vi "Data retrieve engine_SE.vi"(0 "File or Folder Path":path=path "C:/Users/voodoo/Desktop/IV_separat_Vsgsweep_2fields_Vbg-2.8V", 5 "Scan names":string[](array[string]), 7 "IV setup":T3={"# of Vslow"=101, "# Vfast"=41, "#IV Curves at each gate"=1, "B/T offset"=0, "Discard first # curves"=0, "Manual offset"=0, "Field Period"=1, "# of fields/Temperatures"=1}, 9 "index":T2={"A"=3, "B"=4, "C"=2, "D"=4, "E"=3, "N1"=2, "N2"=2, "N3"=3, "N4"=4, "A 1"=8, "A 2"=14, "C 1"=5, "C 2"=1, "E 2"=4}, 11 "Portion of data":cluster{dbl, dbl}(slide)={0.75, 0.25} scale=0.0..1.0, 12 "Decimate point":dbl=1e-10 format="%#_1f", 13 "Extract paramaters from comments?":bool) -> (3 "Comments":string, 4 "IV":cluster{dbl[], dbl[]}[][](array[cluster])=[[{[-2.301174301585294e-09, -2.201174301585294e-09, -2.1011743015852944e-09, -2.0011743015852943e-09, -1.9011743015852942e-09, -1.8011743015852941e-09, -1.701174301585294e-09, -1.601174301585294e-09, -1.5011743015852941e-09, -1.401174301585294e-09, -1.301174301585294e-09, -1.2011743015852942e-09, -1.101174301585294e-09, -1.001174301585294e-09, -9.011743015852942e-10, -8.011743015852941e-10, -7.01174301585294e-10, -6.011743015852942e-10, -5.011743015852941e-10, -4.01174301585294e-10, -3.0117430158529395e-10, -2.0117430158529388e-10, -1.0117430158529423e-10, -1.1743015852941594e-12], [-2.4075285232756958e-05, -1.737972813858452e-05, -1.1037615852397166e-05, -5.267782040080203e-06, 2.4232289247411676e-07, 5.628820057942294e-06, 1.015781505747205e-05, 1.4463328409568988e-05, 1.817222828467457e-05, 2.105509970958606e-05, 2.409775741426245e-05, 2.720796229813868e-05, 3.0197002730537915e-05, 3.3043546244784785e-05, 3.5385544630750595e-05, 3.756777735485851e-05, 3.987253185589809e-05, 4.20620889081888e-05, 4.4006459573108544e-05, 4.587698979226302e-05, 4.7931581768717136e-05, 4.925252522526536e-05, 5.0480327825776546e-05, 8.08077413503745e-08]}]], 6 "IV-2T":cluster{dbl[], dbl[]}[][](array[cluster])=[[{[-2.301174301585294e-09, -2.201174301585294e-09, -2.1011743015852944e-09, -2.0011743015852943e-09, -1.9011743015852942e-09, -1.8011743015852941e-09, -1.701174301585294e-09, -1.601174301585294e-09, -1.5011743015852941e-09, -1.401174301585294e-09, -1.301174301585294e-09, -1.2011743015852942e-09, -1.101174301585294e-09, -1.001174301585294e-09, -9.011743015852942e-10, -8.011743015852941e-10, -7.01174301585294e-10, -6.011743015852942e-10, -5.011743015852941e-10, -4.01174301585294e-10, -3.0117430158529395e-10, -2.0117430158529388e-10, -1.0117430158529423e-10, -1.1743015852941594e-12], [-0.002353462043255516, -0.002297777119659299, -0.002239582947886705, -0.0021846959913649658, -0.0021298090348432263, -0.0020715829478867047, -0.0020166959913649656, -0.0019611544893886803, -0.0019081505368195105, -0.0018609817056506796, -0.0018106102770792509, -0.0017577829478867043, -0.001702609034843226, -0.001644382947886704, -0.001589759034843226, -0.001532834880253854, -0.001467967102476076, -0.0013968026580316317, -0.0013115945420896027, -0.0012138299473531684, -0.00047154515277183454, 0.001680737250983384, 0.0029627659595722446, 4.901687369444213e-06]}]], 8 "Vfast":dbl[][](array[numeric])=[[-1.3]], 10 "Vslow":dbl[](array[numeric])=[-1.3], 14 "N":cluster{"N1":dbl, "N2":dbl, "N3":dbl, "N4":dbl}={"N1"=8999.947, "N2"=0.049942, "N3"=-1.324126602495439e-06, "N4"=0.08912017346699704}, 15 "Vslowest":dbl)   [LabVIEW 2016]
uses:
  <vilib>/addons/WireFlow/_WF_ProgressBar.llb/ProgressBar_WireFlow.lvclass
  <vilib>/Analysis/2dsp.llb/Decimate (single shot, DBL).vi
  <vilib>/Analysis/NI_AALPro.lvlib
panel:
  out "IV 2T 2":cluster{dbl[], dbl[]}(graph)
  out "WF-ProgressBar out":refnum<class "ProgressBar_WireFlow.lvclass">
  in  "Tab Control":T1(tab)
  in  "output array":path[](array[path])
  out "IV 2T":cluster{dbl[], dbl[]}[](graph)=[{[-2.301174301585294e-09, -2.201174301585294e-09, -2.1011743015852944e-09, -2.0011743015852943e-09, -1.9011743015852942e-09, -1.8011743015852941e-09, -1.701174301585294e-09, -1.601174301585294e-09, -1.5011743015852941e-09, -1.401174301585294e-09, -1.301174301585294e-09, -1.2011743015852942e-09, -1.101174301585294e-09, -1.001174301585294e-09, -9.011743015852942e-10, -8.011743015852941e-10, -7.01174301585294e-10, -6.011743015852942e-10, -5.011743015852941e-10, -4.01174301585294e-10, -3.0117430158529395e-10, -2.0117430158529388e-10, -1.0117430158529423e-10, -1.1743015852941594e-12], [-0.002353462043255516, -0.002297777119659299, -0.002239582947886705, -0.0021846959913649658, -0.0021298090348432263, -0.0020715829478867047, -0.0020166959913649656, -0.0019611544893886803, -0.0019081505368195105, -0.0018609817056506796, -0.0018106102770792509, -0.0017577829478867043, -0.001702609034843226, -0.001644382947886704, -0.001589759034843226, -0.001532834880253854, -0.001467967102476076, -0.0013968026580316317, -0.0013115945420896027, -0.0012138299473531684, -0.00047154515277183454, 0.001680737250983384, 0.0029627659595722446, 4.901687369444213e-06]}]
  out "IV":cluster{dbl[], dbl[]}[](graph)=[{[-2.301174301585294e-09, -2.201174301585294e-09, -2.1011743015852944e-09, -2.0011743015852943e-09, -1.9011743015852942e-09, -1.8011743015852941e-09, -1.701174301585294e-09, -1.601174301585294e-09, -1.5011743015852941e-09, -1.401174301585294e-09, -1.301174301585294e-09, -1.2011743015852942e-09, -1.101174301585294e-09, -1.001174301585294e-09, -9.011743015852942e-10, -8.011743015852941e-10, -7.01174301585294e-10, -6.011743015852942e-10, -5.011743015852941e-10, -4.01174301585294e-10, -3.0117430158529395e-10, -2.0117430158529388e-10, -1.0117430158529423e-10, -1.1743015852941594e-12], [-2.4075285232756958e-05, -1.737972813858452e-05, -1.1037615852397166e-05, -5.267782040080203e-06, 2.4232289247411676e-07, 5.628820057942294e-06, 1.015781505747205e-05, 1.4463328409568988e-05, 1.817222828467457e-05, 2.105509970958606e-05, 2.409775741426245e-05, 2.720796229813868e-05, 3.0197002730537915e-05, 3.3043546244784785e-05, 3.5385544630750595e-05, 3.756777735485851e-05, 3.987253185589809e-05, 4.20620889081888e-05, 4.4006459573108544e-05, 4.587698979226302e-05, 4.7931581768717136e-05, 4.925252522526536e-05, 5.0480327825776546e-05, 8.08077413503745e-08]}]
  # "Use to extract gate values in comments\neg. Vsg1="
  # "How many curves at each field/temperature? Usually should be N(Vslow)*N(Vfast)*N(each gate)"
  # "Default:\n4 terminal V vs I \n2 terminal V vs I"
  # "Discard first few IV curves at each gate if the gate need\ntime to settle"
  # "Default decimate on current axis instead of voltage axis. Decimation is needed for extracting dV/dI"
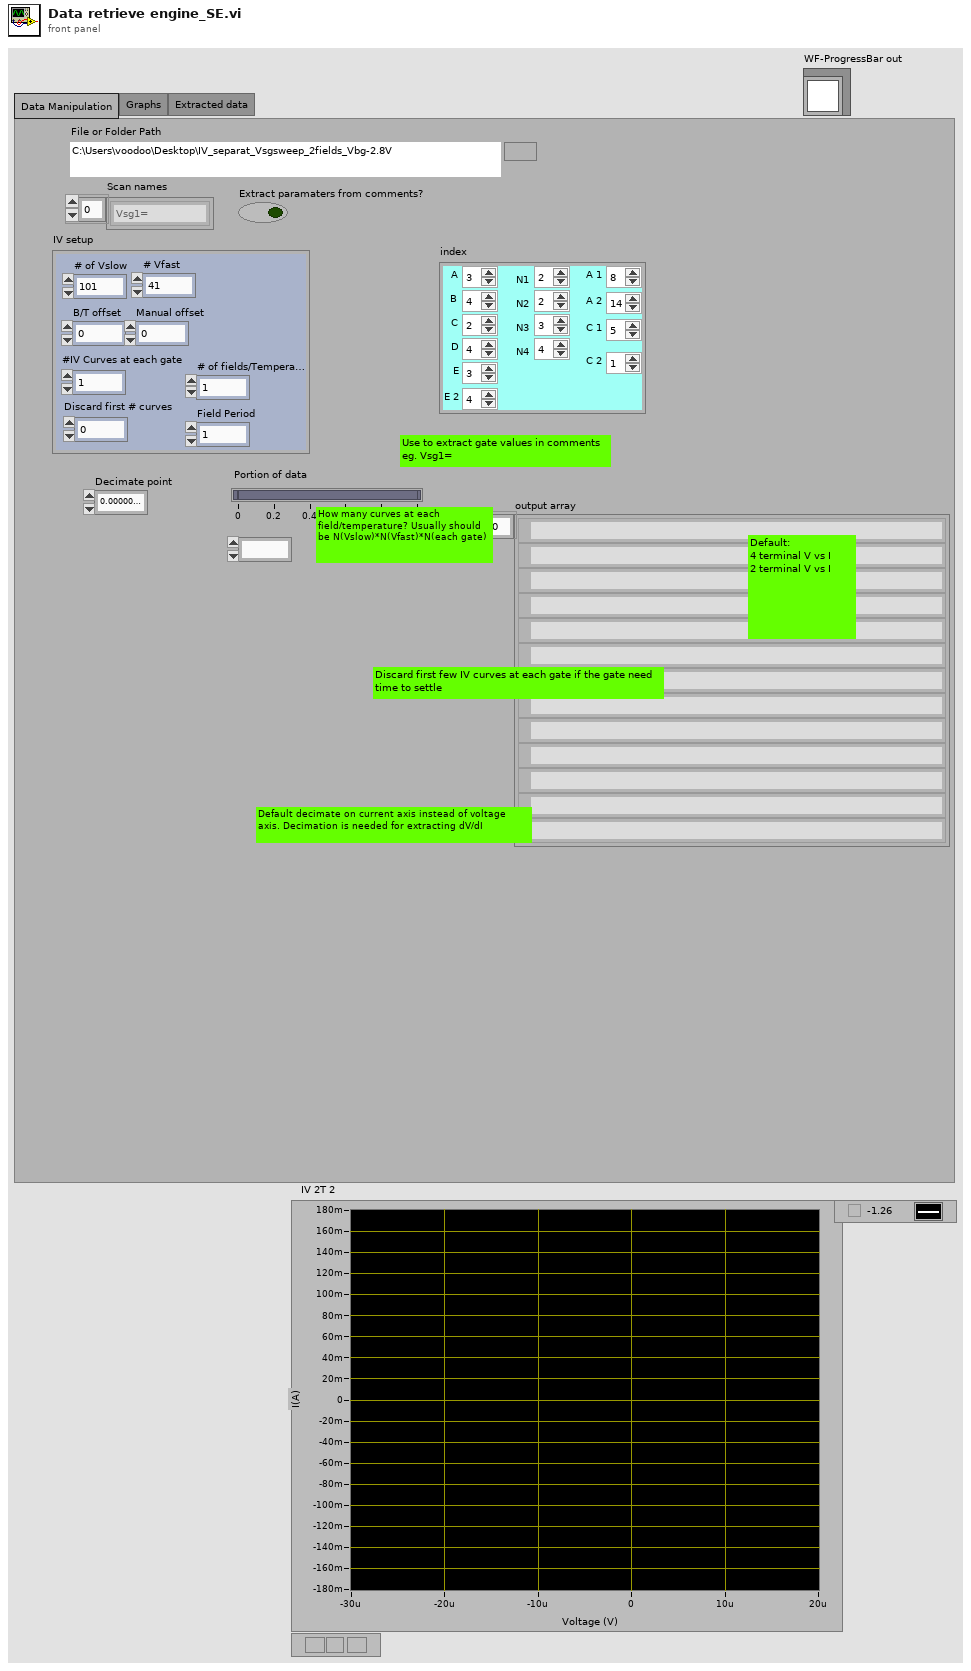
[diagram p1: front panel]
types:
  T1 = enum32{"Data Manipulation", "Graphs", "Extracted data"}
  T2 = cluster{"A":i32, "B":i32, "C":i32, "D":i32, "E":i32, "N1":i32, "N2":i32, "N3":i32, "N4":i32, "A 1":i32, "A 2":i32, "C 1":i32, "C 2":i32, "E 2":i32}
  T3 = cluster{"# of Vslow":i32, "# Vfast":i32, "#IV Curves at each gate":i32, "B/T offset":i32, "Discard first # curves":i32, "Manual offset":i32, "Field Period":i32, "# of fields/Temperatures":i32}
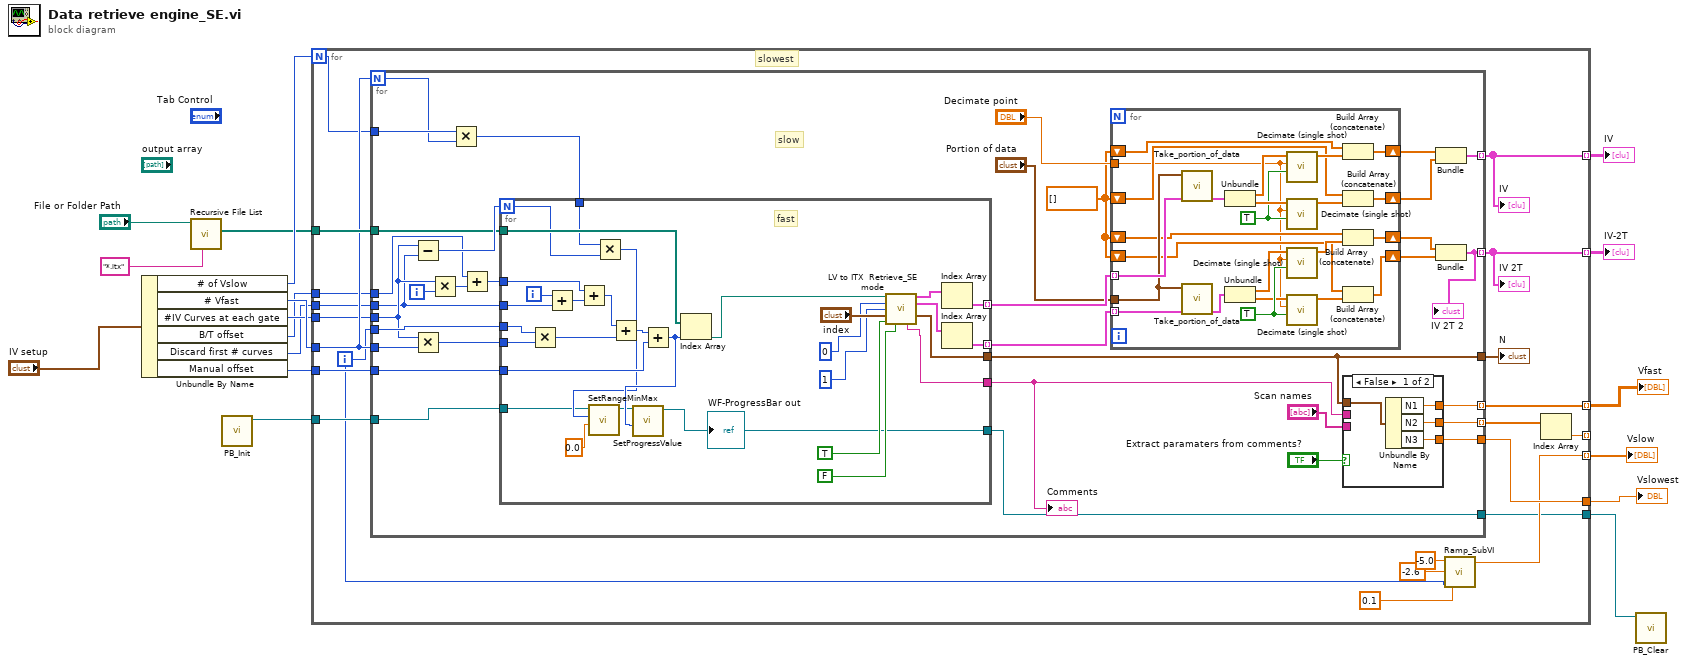
[diagram p0: block diagram]
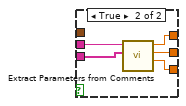
[diagram p2: hidden frame]
diagram:
  n1 = Unbundle By Name("IV setup") -> ("# of Vslow"=w17:i32, "# Vfast"=w16:i32, "#IV Curves at each gate"=w15:i32, "B/T offset"=w13:i32, "Discard first # curves"=w14:i32, "Manual offset"=w12:i32)
  n2 = call <vilib>:"Recursive File List.vi"("pattern"="*.itx", "Folder Path"="File or Folder Path") -> ("All Files in Dir"=w4:path[])  [unwired: 5 in, 4 out]
  n3 = call <vilib>:"PB_Init.vi"() -> ("WF-ProgressBar out"=w5:refnum<class "ProgressBar_WireFlow.lvclass">)  [unwired: 10 in, 1 out]
  n4 = for {
    N: w17 -> [w26]
    tunnel: [w38] -> _ mode=indexing
    tunnel: w4 -> [w36]
    tunnel: w16 -> [w35]
    tunnel: w15 -> [w34]
    tunnel: w14 -> [w33]
    tunnel: w13 -> [w32]
    tunnel: w12 -> [w31]
    tunnel: [w30] -> w11 mode=indexing
    tunnel: [w29] -> w10 mode=indexing
    tunnel: [w27] -> w9 mode=indexing
    tunnel: [w20] -> w8
    tunnel: w5 -> [w25]
    tunnel: [w19] -> w3 mode=indexing
    tunnel: [w18] -> w1
    i -> [w21]
    # "slowest"
    n5 = for {
      N: w35 -> [w43]
      tunnel: w35 -> [w69]
      tunnel: w21 -> [w68]
      tunnel: [w48] -> w37
      tunnel: w36 -> [w66]
      tunnel: w34 -> [w65]
      tunnel: w33 -> [w64]
      tunnel: w32 -> [w63]
      tunnel: w31 -> [w62]
      tunnel: [w40] -> w29 mode=indexing
      tunnel: [w52] -> w30 mode=indexing
      tunnel: [w45] -> w20
      tunnel: [w51] -> w28 mode=indexing
      tunnel: [w46] -> w27 mode=indexing
      tunnel: w26 -> [w44]
      tunnel: w25 -> [w41]
      tunnel: [w39] -> w18
      i -> [w72]
      w55 = dbl[] []
      # "slow"
      n6 = Subtract(x=w65, y=w64) -> (x-y=w67:i32)
      n7 = Multiply(x=w65, y=w69) -> (x*y=w70:i32)
      n8 = Multiply(x=w65, y=w72) -> (x*y=w73:i32)
      n9 = Multiply(x=w44, y=w43) -> (x*y=w42:i32)
      n10 = Add(x=w63, y=w73) -> (x+y=w71:i32)
      n11 = for {
        N: w67 -> [w112]
        tunnel: w71 -> [w137]
        tunnel: [w116] -> w49
        tunnel: w70 -> [w134]
        tunnel: [w133] -> w61 mode=indexing
        tunnel: w68 -> [w131]
        tunnel: [w117] -> w48
        tunnel: w64 -> [w130]
        tunnel: [w129] -> w60 mode=indexing
        tunnel: w66 -> [w128]
        tunnel: w62 -> [w126]
        tunnel: w42 -> [w113]
        tunnel: w41 -> [w110]
        tunnel: [w107] -> w39
        i -> [w115]
        # "fast"
        n12 = Multiply(x=w131, y=w134) -> (x*y=w135:i32)
        n13 = Add(x=w115, y=w130) -> (x+y=w132:i32)
        n14 = Add(x=w137, y=w132) -> (x+y=w136:i32)
        n15 = Multiply(x=w113, y=w112) -> (x*y=w111:i32)
        n16 = call-dynamic "SetRangeMinMax.vi"("Min (0)"=0.0, "Max (1)"=w111, "WF-ProgressBar in"=w110) -> ("WF-ProgressBar out"=w108:refnum<class "ProgressBar_WireFlow.lvclass">)  [unwired: 7 in, 1 out]
        n17 = Add(x=w136, y=w135) -> (x+y=w127:i32)
        n18 = Add(x=w127, y=w126) -> (x+y=w114:i32)
        n19 = call-dynamic "SetProgressValue.vi"("Value"=w114, "WF-ProgressBar in"=w108) -> ("WF-ProgressBar out"=w107:refnum<class "ProgressBar_WireFlow.lvclass">)  [unwired: 7 in, 2 out]
        "WF-ProgressBar out" <- w107
        n20 = Index Array(array=w128, index=w114) -> (element=w122:path)
        n21 = call "LV to ITX  Retrieve_SE mode.vi"("File or Folder Path"=w122, "offset"=0, "length"=1, "index"="index", "stop"=TRUE, "file contains 2D data?"=FALSE ("List folder?")) -> ("A vs B"=w125:cluster{dbl[], dbl[]}[], "C vs D"=w124:cluster{dbl[], dbl[]}[], "N"=w117:cluster{"N1":dbl, "N2":dbl, "N3":dbl, "N4":dbl}, "Comments"=w116:string)  [unwired: 6 out]
        n22 = Index Array(array=w125) -> (element=w133:cluster{dbl[], dbl[]})  [unwired: 1 in]
        n23 = Index Array(array=w124) -> (element=w129:cluster{dbl[], dbl[]})  [unwired: 1 in]
      }
      "Comments" <- w49
      n24 = for {
        tunnel: w61 -> [w106] mode=indexing
        tunnel: w60 -> [w89] mode=indexing
        tunnel: "Portion of data" -> [w88]
        tunnel: "Decimate point" -> [w83]
        shift-right: [w101] -> w57
        shift-left: w55 -> [w99]
        shift-right: [w97] -> w56
        shift-left: w55 -> [w96]
        shift-right: [w87] -> w54
        shift-left: w55 -> [w86]
        shift-right: [w85] -> w53
        shift-left: w55 -> [w84]
        w92 = TRUE ("averaging")
        w103 = TRUE ("averaging")
        n25 = call <userlib>:"Take_portion_of_data.vi"("input IV"=w106, "Slide"=w88) -> ("Output IV"=w102:cluster{dbl[], dbl[]})  [unwired: 5 in]
        n26 = call <userlib>:"Take_portion_of_data.vi"("input IV"=w89, "Slide"=w88) -> ("Output IV"=w93:cluster{dbl[], dbl[]})  [unwired: 5 in]
        n27 = Unbundle(w102) -> (w104:dbl[], w105:dbl[])
        n28 = Unbundle(w93) -> (w91:dbl[], w90:dbl[])
        n29 = call-poly <vilib>:"Decimate (single shot).vi"("averaging"=w103, "decimating factor"=w83, "X"=w104) -> ("Decimated Array"=w100:dbl[])  [unwired: 7 in, 1 out]
        n30 = call-poly <vilib>:"Decimate (single shot).vi"("averaging"=w103, "decimating factor"=w83, "X"=w105) -> ("Decimated Array"=w98:dbl[])  [unwired: 7 in, 1 out]
        n31 = call-poly <vilib>:"Decimate (single shot).vi"("averaging"=w92, "decimating factor"=w83, "X"=w91) -> ("Decimated Array"=w94:dbl[])  [unwired: 7 in, 1 out]
        n32 = call-poly <vilib>:"Decimate (single shot).vi"("averaging"=w92, "decimating factor"=w83, "X"=w90) -> ("Decimated Array"=w95:dbl[])  [unwired: 7 in, 1 out]
        n33 = Build Array (concatenate)(w99, w100) -> (w101:dbl[])
        n34 = Build Array (concatenate)(w96, w98) -> (w97:dbl[])
        n35 = Build Array (concatenate)(w86, w94) -> (w87:dbl[])
        n36 = Build Array (concatenate)(w84, w95) -> (w85:dbl[])
      }
      n37 = case shown="False" "Extract paramaters from comments?" {
        tunnel: [w74 w82] -> w46
        tunnel: [w75 w81] -> w45
        tunnel: [w76 w80] -> w51
        tunnel: "Scan names" -> [_ w79]
        tunnel: w49 -> [_ w78]
        tunnel: w48 -> [w77 _]
        frame False {
          n38 = Unbundle By Name(w77) -> ("N1"=w74:dbl, "N2"=w76:dbl, "N3"=w75:dbl)
        }
        frame True {
          n39 = call <userlib>:"Extract Parameters from Comments.vi"("Scan names"=w79, "Comments"=w78) -> ("Numeric"=w81:dbl, "Numeric 3"=w80:dbl, "Numeric 2"=w82:dbl)  [unwired: 7 in]
        }
      }
      n40 = Bundle(w57, w56) -> (w52:cluster{dbl[], dbl[]})  [unwired: 1 in]
      n41 = Bundle(w54, w53) -> (w40:cluster{dbl[], dbl[]})  [unwired: 1 in]
      "IV 2T 2" <- w40
    }
    "IV" <- w30
    "N" <- w37
    "IV 2T" <- w29
    n42 = call <userlib>:"Ramp_SubVI.vi"("index"=w21, "step"=0.1, "end"=-2.6, "start"=-5.0) -> ("Numeric"=w19:dbl)  [unwired: 1 in, 1 out]
    n43 = Index Array(array=w28) -> (element=w38:dbl)  [unwired: 1 in]
  }
  "Vslow" <- w3
  "Vfast" <- w9
  "IV" <- w11
  "IV-2T" <- w10
  "Vslowest" <- w8
  n44 = call-dynamic "PB_Clear.vi"("WF-ProgressBar in"=w1) -> ()  [unwired: 9 in, 2 out]
